vi "XML Script - Coordinate String.vi"(1 "y":i32=-1, 2 "x":i32=-1) -> (0 "(x,y)":string)   [LabVIEW 2017]
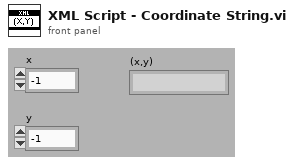
[diagram p1: front panel]
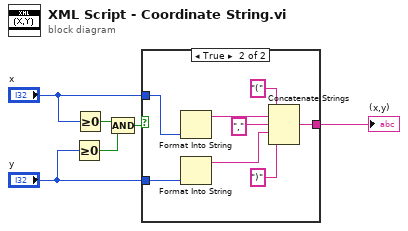
[diagram p0: block diagram]
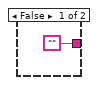
[diagram p2: hidden frame]
diagram:
  n1 = Greater Or Equal To 0?(x="y") -> (x >= 0?=w3:bool)
  n2 = Greater Or Equal To 0?(x="x") -> (x >= 0?=w2:bool)
  n3 = Compound Arithmetic op=AND(w2, w3) -> (w1:bool)
  n4 = case shown="True" w1 {
    tunnel: "x" -> [_ w15]
    tunnel: "y" -> [_ w14]
    tunnel: ["" w8] -> w6
    frame False {
    }
    frame True {
      n5 = Format Into String(w15) -> (resulting string=w12:string)  [unwired: 3 in, 1 out]
      n6 = Format Into String(w14) -> (resulting string=w10:string)  [unwired: 3 in, 1 out]
      n7 = Concatenate Strings("(", w12, ",", w10, ")") -> (w8:string)
    }
  }
  "(x,y)" <- w6
